vi "Ex3.vi"() -> ()   [LabVIEW 2019]
panel:
  out "Error":bool
  out "Nom":string
  out "Prénom":string
  in  "Nom brut":string
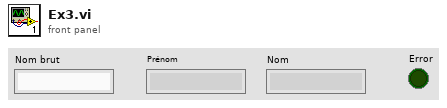
[diagram p1: front panel]
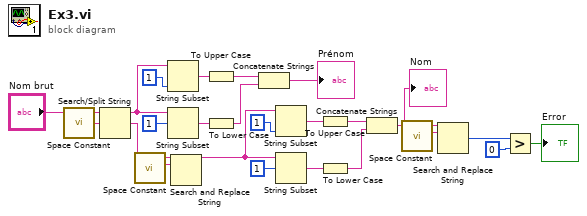
[diagram p0: block diagram]
diagram:
  n1 = call <vilib>:"Space Constant.vi"() -> ("String"=w23:string)
  n2 = Search/Split String(string="Nom brut", search string/char (-)=w23) -> (substring before match=w19:string, match + rest of string=w21:string)  [unwired: 1 in, 1 out]
  n3 = call <vilib>:"Space Constant.vi"() -> ("String"=w22:string)
  n4 = String Subset(string=w19, length (rest)=1) -> (substring=w17:string)  [unwired: 1 in]
  n5 = String Subset(string=w19, offset (0)=1) -> (substring=w9:string)  [unwired: 1 in]
  n6 = Search and Replace String(input string=w21, search string=w22) -> (result string=w11:string)  [unwired: 6 in, 3 out]
  n7 = To Upper Case(1:w17) -> (0:w16:string)
  n8 = To Lower Case(string=w9) -> (all lower case string=w8:string)
  n9 = Concatenate Strings(w16, w8) -> (→"Prénom":string)
  n10 = String Subset(string=w11, length (rest)=1) -> (substring=w13:string)  [unwired: 1 in]
  n11 = String Subset(string=w11, offset (0)=1) -> (substring=w7:string)  [unwired: 1 in]
  n12 = To Upper Case(1:w13) -> (0:w12:string)
  n13 = To Lower Case(string=w7) -> (all lower case string=w6:string)
  n14 = Concatenate Strings(w12, w6) -> (w4:string)
  "Nom" <- w4
  n15 = call <vilib>:"Space Constant.vi"() -> ("String"=w5:string)
  n16 = Search and Replace String(input string=w4, search string=w5) -> (number of replacements=w3:i32)  [unwired: 6 in, 3 out]
  n17 = Greater?(x=w3, y=0) -> (0:→"Error":bool)
